vi "Init from Size.vi"(8 "error in (no error)":errorcluster, 10 "size":dbl, 11 "Cave  in":refnum<class "Cave.lvclass">) -> (0 "error out":errorcluster, 3 "Cave out":refnum<class "Cave.lvclass">)   [LabVIEW 2021, in "d15.lvlib" / "Cave.lvclass"]
uses:
  Cave.lvclass
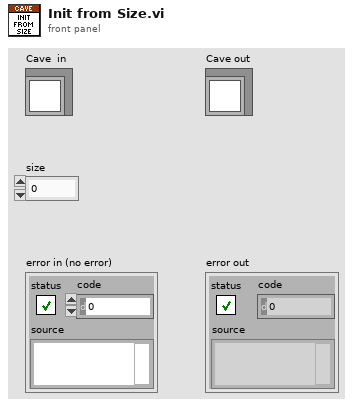
[diagram p1: front panel]
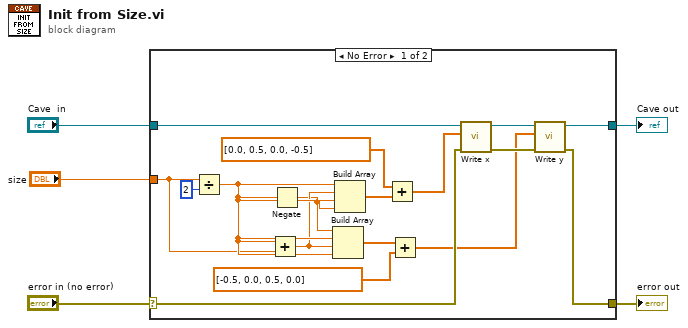
[diagram p0: block diagram]
diagram:
  n1 = case shown="No Error" "error in (no error)" {
    selector: "error in (no error)" -> [w16 w24]
    tunnel: [w13 w24] -> w4
    tunnel: [w15 w23] -> w2
    tunnel: "Cave  in" -> [w19 w23]
    tunnel: "size" -> [w20 _]
    frame No Error {
      n2 = Divide(x=w20, y=2) -> (x/y=w21:dbl)
      n3 = Add(x=w21, y=w20) -> (x+y=w11:dbl)
      n4 = Negate(x=w21) -> (-x=w10:dbl)
      n5 = Build Array(w10, w21, w11, w21) -> (w12:dbl[])
      n6 = Build Array(w21, w11, w21, w10) -> (w17:dbl[])
      n7 = Add(x=dbl[] [0.0, 0.5, 0.0, -0.5], y=w17) -> (x+y=w9:dbl[])
      n8 = Add(x=w12, y=dbl[] [-0.5, 0.0, 0.5, 0.0]) -> (x+y=w7:dbl[])
      n9 = call-dynamic "Write x.vi"("error in (no error)"=w16, "x"=w9, "Diamond in"=w19) -> ("error out"=w14:errorcluster, "Diamond out"=w18:refnum<class "Cave.lvclass">)  [unwired: 7 in]
      n10 = call-dynamic "Write y.vi"("error in (no error)"=w14, "y"=w7, "Diamond in"=w18) -> ("error out"=w13:errorcluster, "Diamond out"=w15:refnum<class "Cave.lvclass">)  [unwired: 7 in]
    }
    frame Error {
    }
  }
  "error out" <- w4
  "Cave out" <- w2
